vi "CWD.vi"(8 "error in (no error)":errorcluster, 10 "RemoteDirectory":string, 11 "FTP in":refnum<class "FTP.lvclass">) -> (0 "error out":errorcluster, 3 "FTP out":refnum<class "FTP.lvclass">)   [LabVIEW 2017, in "FTP_UpgradeCSMF.lvlib" / "FTP.lvclass"]
uses:
  FTP.lvclass
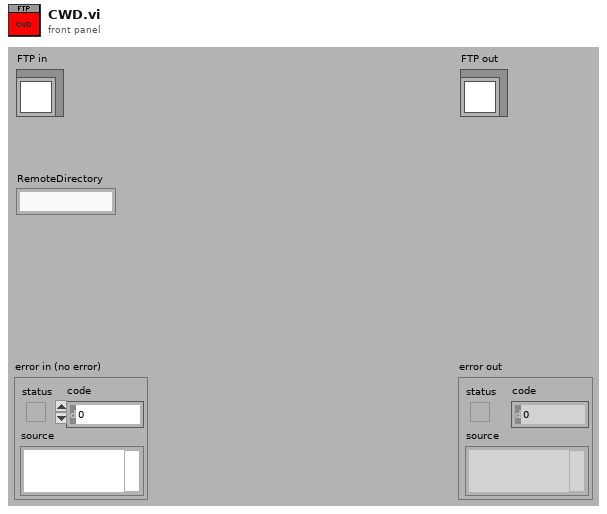
[diagram p1: front panel]
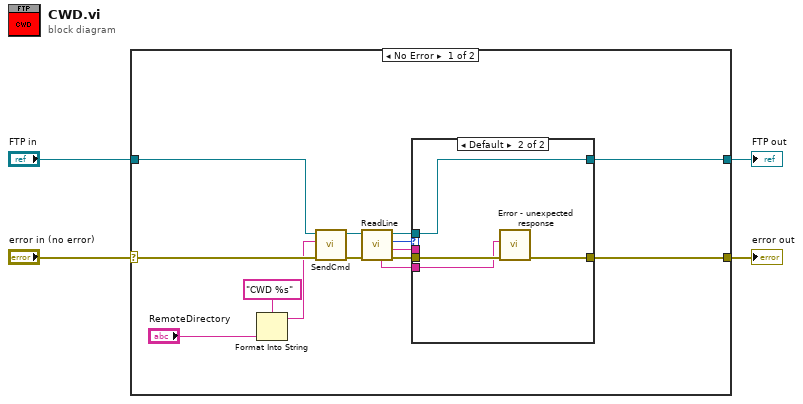
[diagram p0: block diagram]
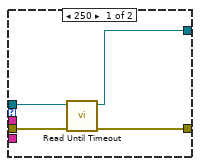
[diagram p2: hidden frame]
diagram:
  n1 = case shown="No Error" "error in (no error)" {
    selector: "error in (no error)" -> [w11 w28]
    tunnel: [w10 w28] -> w3
    tunnel: [w9 w27] -> w1
    tunnel: "FTP in" -> [w12 w27]
    frame No Error {
      n2 = Format Into String(format string="CWD %s", "RemoteDirectory") -> (resulting string=w8:string)  [unwired: 2 in, 1 out]
      n3 = call "SendCmd.vi"("error in (no error)"=w11, "cmd"=w8, "FTP in"=w12) -> ("error out"=w18:errorcluster, "FTP out"=w17:refnum<class "FTP.lvclass">)  [unwired: 7 in]
      n4 = call "ReadLine.vi"("error in (no error)"=w18, "FTP in"=w17) -> ("error out"=w14:errorcluster, "Line"=w13:string, "code"=w15:i32, "FTP out"=w16:refnum<class "FTP.lvclass">, "Full Line"=w5:string)  [unwired: 5 in]
      n5 = case shown="Default" w15 {
        tunnel: w16 -> [w21 w26]
        tunnel: w14 -> [w22 w25]
        tunnel: [w20 w24] -> w10
        tunnel: [w19 w26] -> w9
        tunnel: w13 -> [_ _]
        tunnel: w5 -> [_ w23]
        frame 250 {
          n6 = call "Read Until Timeout.vi"("error in (no error)"=w22, "FTP in"=w21) -> ("error out"=w20:errorcluster, "FTP out"=w19:refnum<class "FTP.lvclass">)  [unwired: 8 in]
        }
        frame Default {
          n7 = call "Error - unexpected response.vi"("error in (no error)"=w25, "Full Response"=w23) -> ("error out"=w24:errorcluster)  [unwired: 9 in]
        }
      }
    }
    frame Error {
    }
  }
  "error out" <- w3
  "FTP out" <- w1
